vi "Convert ASCII to Hex.vi"(0 "String In":string) -> (1 "Hex ASCII String Length":i32, 2 "Hex ASCII String Out":string)   [LabVIEW 2024, in "Bronkhorst FLOW-BUS.lvlib"]
doc: "Converts a normal ASCII string to the format expected by the FLOW-BUS instrument. The Hex Value of the ASCII characters gets converted to their ASCII values (e.g. the input string \"Air\" becomes \"416972\")."
uses:
  Bronkhorst FLOW-BUS.lvlib
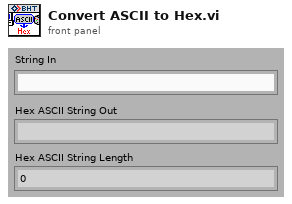
[diagram p1: front panel]
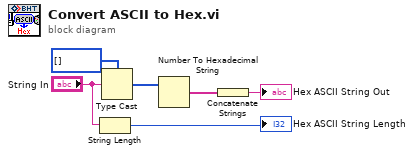
[diagram p0: block diagram]
diagram:
  n1 = String Length(string="String In") -> (length=→"Hex ASCII String Length":i32)
  n2 = Type Cast(type=u8[] [], x="String In") -> (*(type *) &x=w1:u8[])
  n3 = Number To Hexadecimal String(2:w1) -> (0:w3:string[])  [unwired: 1 in]
  n4 = Concatenate Strings(w3) -> (→"Hex ASCII String Out":string)
